vi "Close.vi"(8 "error in (no error)":errorcluster, 11 "GPIB in":refnum<class "GPIB.lvclass">) -> (0 "error out":errorcluster, 3 "GPIB out":refnum<class "GPIB.lvclass">)   [LabVIEW 2013, in "GPIB.lvclass"]
uses:
  GPIB.lvclass
  VISA/VISA.lvclass/VISA.ctl
  VISA/Read Ref.vi
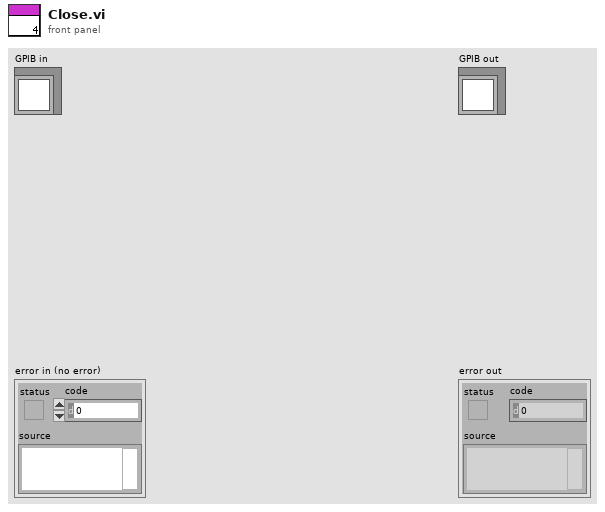
[diagram p1: front panel]
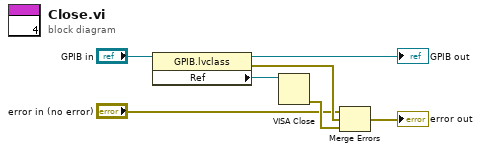
[diagram p0: block diagram]
diagram:
  n1 = property class="GPIB.lvclass"(reference="GPIB in") -> (reference out=→"GPIB out":refnum<class "GPIB.lvclass">, error out=w5:errorcluster, "Ref"=w7:refnum<visa-resource-name>)  [unwired: 1 in]
  n2 = VISA Close(VISA resource name=w7) -> (error out=w6:errorcluster)  [unwired: 1 in]
  n3 = Merge Errors("error in (no error)", w5, w6) -> (→"error out":errorcluster)
